vi "PAN_DBS_parse_request.vi"(8 "error in (no error)":errorcluster, 10 "desired point":string, 11 "Database RefNum in":T1) -> (0 "number of points":i32, 1 "mult. points?":bool, 2 "names":string[](array[string]), 3 "found":bool, 4 "error out":errorcluster)   [LabVIEW 2016]
uses:
  Modules/DBSHAND/private/vis/DatabaseHand_RefNum.ctl
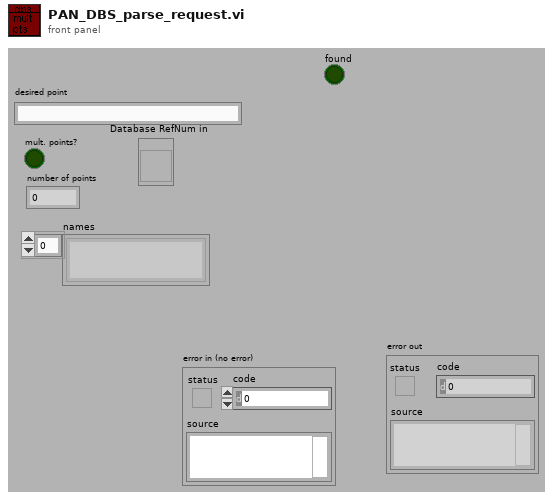
[diagram p1: front panel]
types:
  T1 = typedef "DatabaseHand_RefNum.ctl" = refnum<vi>
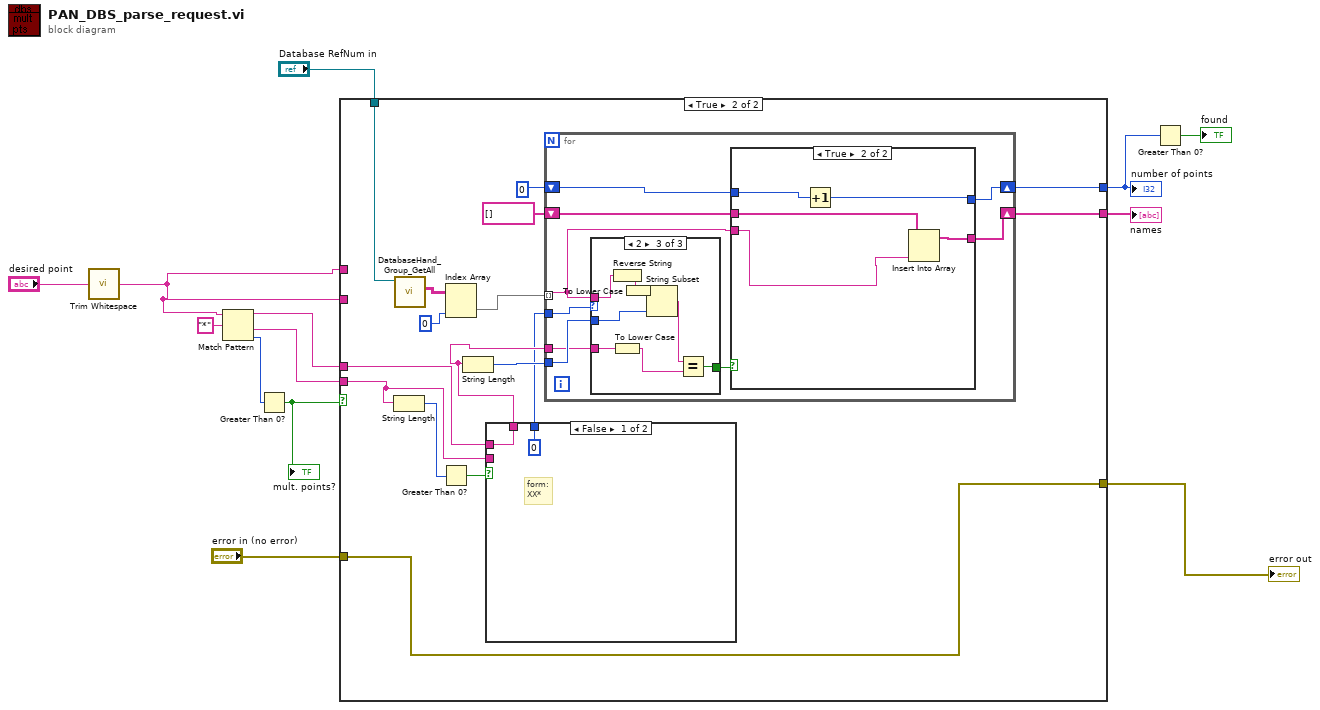
[diagram p0: block diagram]
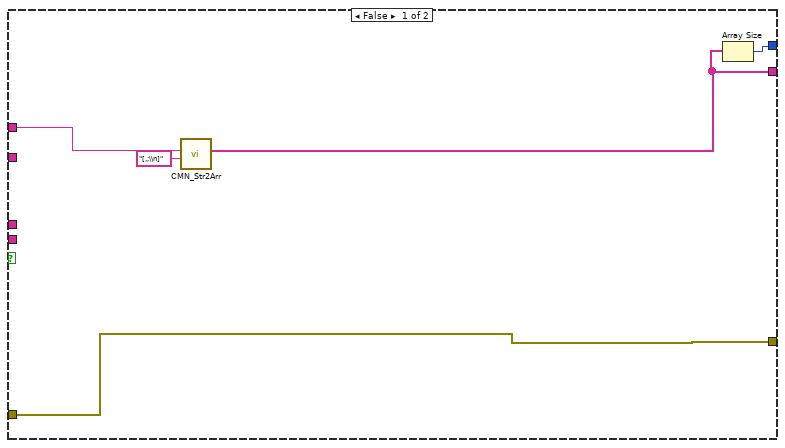
[diagram p2: hidden frame]
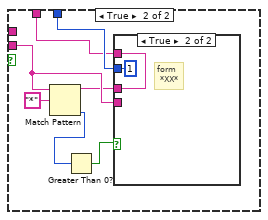
[diagram p3: hidden frame]
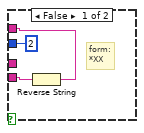
[diagram p4: hidden frame]
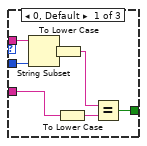
[diagram p5: hidden frame]
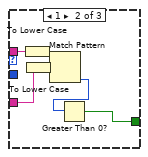
[diagram p6: hidden frame]
diagram:
  n1 = call <vilib>:"Trim Whitespace.vi"("string"="desired point") -> ("trimmed string"=w1:string)  [unwired: 1 in]
  n2 = Match Pattern(string=w1, regular expression="*") -> (before substring=w10:string, after substring=w8:string, offset past match=w12:i32)  [unwired: 2 out]
  n3 = Greater Than 0?(x=w12) -> (x > 0?=w11:bool)
  "mult. points?" <- w11
  n4 = case shown="True" w11 {
    tunnel: w10 -> [_ w26]
    tunnel: [w18 w31] -> w7
    tunnel: [w16 w30] -> w9
    tunnel: w8 -> [_ w27]
    tunnel: w1 -> [_ _]
    tunnel: "error in (no error)" -> [w14 w23]
    tunnel: [w14 w23] -> w4
    tunnel: w1 -> [w17 _]
    tunnel: "Database RefNum in" -> [_ w22]
    frame False {
      n5 = call "CMN_Str2Arr.vi"("separator"="[,;\\n]", "string in"=w17) -> ("Array out"=w16:string[])  [unwired: 2 in, 7 out]
      n6 = Array Size(array=w16) -> (size(s)=w18:i32)
    }
    frame True {
      n7 = String Length(string=w27) -> (length=w29:i32)
      n8 = call "DatabaseHand_Group_GetAll.vi"("Database RefNum in"=w22) -> ("database array"=w21:string[][])  [unwired: 1 in, 9 out]
      n9 = Greater Than 0?(x=w29) -> (x > 0?=w28:bool)
      n10 = Index Array(array=w21, index (col)=0 ("index (row)")) -> (element=w20:string[])  [unwired: 1 in]
      n11 = case shown="False" w28 {
        tunnel: w27 -> [_ w39]
        tunnel: w26 -> [w36 _]
        tunnel: [w36 w37] -> w25
        tunnel: [0 w40] -> w24
        frame False {
          # "form:\nXX*"
        }
        frame True {
          n12 = Match Pattern(string=w39, regular expression="*") -> (before substring=w38:string, offset past match=w42:i32)  [unwired: 3 out]
          n13 = Greater Than 0?(x=w42) -> (x > 0?=w41:bool)
          n14 = case shown="True" w41 {
            tunnel: [2 1] -> w40
            tunnel: w39 -> [w45 _]
            tunnel: w38 -> [_ w47]
            tunnel: [w44 w47] -> w37
            frame False {
              # "form:\n*XX"
              n15 = Reverse String(1:w45) -> (0:w44:string)
            }
            frame True {
              # "form\n *XX*"
            }
          }
        }
      }
      n16 = String Length(string=w25) -> (length=w34:i32)
      n17 = for {
        tunnel: w25 -> [w56]
        tunnel: w20 -> [w54] mode=indexing
        tunnel: w34 -> [w57]
        shift-right: [w52] -> w31
        shift-left: 0 -> [w53]
        shift-right: [w51] -> w30
        shift-left: string[] [] -> [w50]
        tunnel: w24 -> [w49]
        n18 = case shown="2" w49 {
          tunnel: w57 -> [w64 _ w76]
          tunnel: w56 -> [w63 w69 w74]
          tunnel: [w62 w67 w73] -> w55
          tunnel: w54 -> [w60 w70 w78]
          frame 0, Default {
            n19 = String Subset(string=w60, length (rest)=w64) -> (substring=w61:string)  [unwired: 1 out]
            n20 = To Lower Case(string=w61) -> (all lower case string=w59:string)
            n21 = To Lower Case(string=w63) -> (all lower case string=w58:string)
            n22 = Equal?(x=w59, y=w58) -> (x = y?=w62:bool)
          }
          frame 1 {
            n23 = To Lower Case(string=w70) -> (all lower case string=w66:string)
            n24 = To Lower Case(string=w69) -> (all lower case string=w65:string)
            n25 = Match Pattern(string=w66, regular expression=w65) -> (offset past match=w68:i32)  [unwired: 4 out]
            n26 = Greater Than 0?(x=w68) -> (x > 0?=w67:bool)
          }
          frame 2 {
            n27 = Reverse String(1:w78) -> (0:w77:string)
            n28 = To Lower Case(string=w74) -> (all lower case string=w71:string)
            n29 = To Lower Case(string=w77) -> (all lower case string=w72:string)
            n30 = String Subset(string=w72, length (rest)=w76) -> (substring=w75:string)  [unwired: 1 out]
            n31 = Equal?(x=w75, y=w71) -> (x = y?=w73:bool)
          }
        }
        n32 = case shown="True" w55 {
          tunnel: w54 -> [_ w81]
          tunnel: w53 -> [w80 w85]
          tunnel: [w80 w84] -> w52
          tunnel: [w79 w83] -> w51
          tunnel: w50 -> [w79 w82]
          frame False {
          }
          frame True {
            n33 = Increment(x=w85) -> (x+1=w84:i32)
            n34 = Insert Into Array(array=w82, new element=w81) -> (w83:string[])  [unwired: 1 in]
          }
        }
      }
    }
  }
  "number of points" <- w7
  "names" <- w9
  "error out" <- w4
  n35 = Greater Than 0?(x=w7) -> (x > 0?=→"found":bool)
